vi "PROG 3 - Sum of Two Numbers.vi"() -> ()   [LabVIEW 2012]
panel:
  out "Thermometer":dbl(slide) scale=0.0..500.0
  out "The Sum of The Two Numbers is":dbl
  in  "Numeric 2":dbl
  in  "Numeric 1":dbl
  # "Numeric Indicator"
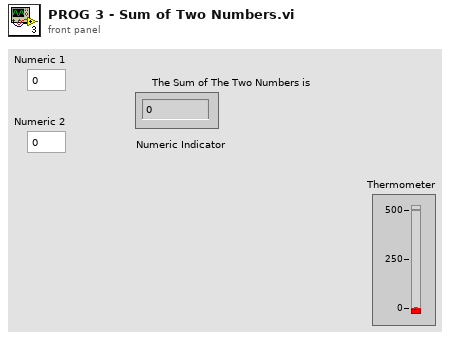
[diagram p1: front panel]
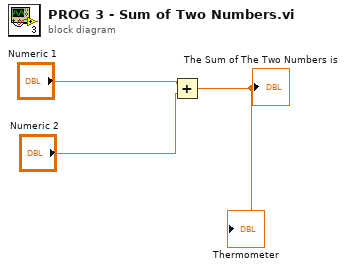
[diagram p0: block diagram]
diagram:
  n1 = Add(x="Numeric 1", y="Numeric 2") -> (x+y=→"The Sum of The Two Numbers is" →"Thermometer":dbl)
